vi "niFpgaReadControlTemplate.vi"(0 "reference":refnum<vi>, 5 "Control Name":string, 7 "Value in":variant, 11 "error in (no error)":errorcluster) -> (8 "Value":variant, 15 "error out":errorcluster)   [LabVIEW 2017]
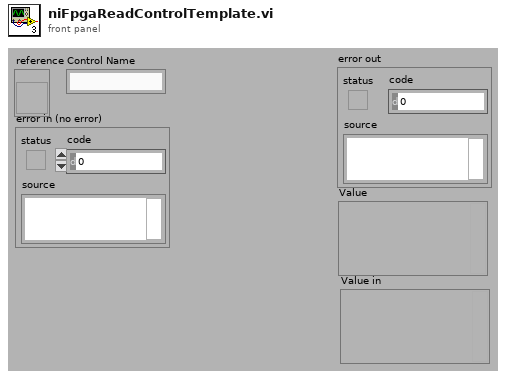
[diagram p1: front panel]
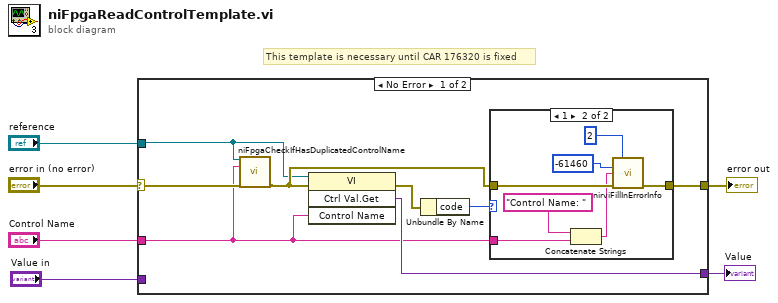
[diagram p0: block diagram]
diagram:
  # "This template is necessary until CAR 176320 is fixed"
  n1 = case shown="No Error" "error in (no error)" {
    selector: "error in (no error)" -> [w10 w23]
    tunnel: "reference" -> [w8 _]
    tunnel: [w14 _] -> w5
    tunnel: "Control Name" -> [w7 _]
    tunnel: [w11 w23] -> w3
    tunnel: "Value in" -> [_ _]
    frame No Error {
      n2 = call <vilib>:"niFpgaCheckIfHasDuplicatedControlName.vi"("reference"=w8, "Control Name"=w7, "error in (no error)"=w10) -> ("error out"=w9:errorcluster)  [unwired: 12 in]
      n3 = invoke class="VI" method="Ctrl Val.Get"(reference=w8, error in=w9, "Control Name"=w7) -> (error out=w12:errorcluster, "Get Control Value Variant"=w14:variant)  [unwired: 1 in, 2 out]
      n4 = Unbundle By Name(w12) -> ("code"=w13:i32)
      n5 = case shown="1" w13 {
        tunnel: w9 -> [w15 w22]
        tunnel: [w15 w21] -> w11
        tunnel: w7 -> [_ w18]
        frame Default {
        }
        frame 1 {
          n6 = Concatenate Strings("Control Name: " ("extended error info"), w18) -> (w17:string)
          n7 = call <vilib>:"nirviFillInErrorInfo.vi"("depth"=2, "status code"=-61460, "extended error info"=w17, "error in"=w22) -> ("error out"=w21:errorcluster)  [unwired: 11 out]
        }
      }
    }
    frame Error {
    }
  }
  "error out" <- w3
  "Value" <- w5
